vi "DataFlowProgrammingBasics.vi"() -> ()   [LabVIEW 2018]
panel:
  in  "Slide":dbl(slide) scale=0.0..200.0
  out "Thermometer":dbl(slide) scale=0.0..100.0
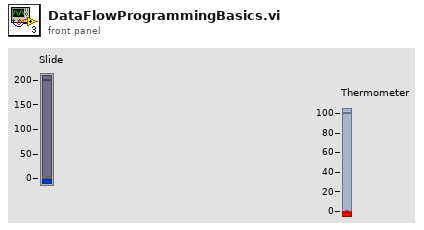
[diagram p1: front panel]
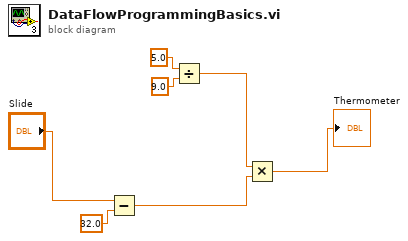
[diagram p0: block diagram]
diagram:
  n1 = Subtract(x="Slide", y=32.0) -> (x-y=w6:dbl)
  n2 = Divide(x=5.0, y=9.0) -> (x/y=w5:dbl)
  n3 = Multiply(x=w5, y=w6) -> (x*y=→"Thermometer":dbl)
